vi "SV Aures Sharpness (Octave_2014) (1 Ch).vi"(0 "octave spectrum":T7={"nominal frequencies [Hz]"=[25.0, 31.5, 40.0, 50.0, 63.0, 80.0, 100.0, 125.0, 160.0, 200.0, 250.0, 315.0, 400.0, 500.0, 630.0, 800.0, 1000.0, 1250.0, 1600.0, 2000.0, 2500.0, 3150.0, 4000.0, 5000.0, 6300.0, 8000.0, 10000.0, 12500.0], "band power"=[-99.0, -99.0, -99.0, -99.0, -99.0, -99.0, -99.0, -99.0, -99.0, -99.0, -99.0, -99.0, -99.0, -99.0, 20.0, 40.0, 60.0, 40.0, 20.0, -99.0, -99.0, -99.0, -99.0, -99.0, -99.0, -99.0, -99.0, -99.0]} {"band power" format="%.2f"; "nominal frequencies [Hz]" format="%.2f"}, 1 "diffuse field":bool, 9 "octave info":T2={"standard"=enum."IEC 61260", "bandwidth"=enum."1/3 octave", "low band"=-16, "high band"=11, "weighting filter"=0, "dB reference"=2e-05, "dB On"=TRUE, "unit label"="Pa^2 rms|SV Units|dB ref 20u Pa", "channel name"="", "description"="", "engineering units"=2, "custom label"="", "spectrum type"=enum."power", "spectral density"=FALSE, "filters settled"=FALSE} {"engineering units" items=["custom..."=0, "V"=1, "A"=21, "C"=30, "pC"=31, "s"=32, "-"=29, "Pa"=2, "N"=20, "g"=3, "m/s^2"=4, "m/s"=5, "m"=6, "mm/s"=12, "mm"=13, "micron/s"=14, "micron"=15, "in/s^2"=7, "in/s"=8, "in"=9, "mil/s"=10, "mil"=11, "rad/s^2"=16, "rad/s"=17, "rad"=18, "deg/s^2"=26, "deg/s"=27, "deg"=28, "RPM"=22, "cycle/s^2"=23, "Hz"=24, "cycle"=25, "strain"=19]; "dB reference" format="%.2e"; "weighting filter" items=["Linear", "A-weighting", "B-weighting", "C-weighting", "ITU-R 468-4", "Dolby", "CCITT", "C-message", "Wb", "Wc", "Wd", "We", "Wf", "Wh", "Wj", "Wk", "Wm", "AES17 20 kHz lowpass", "AES17 40 kHz lowpass", "AES17 20 kHz highpass", "AES17 40 kHz highpass"]}, 11 "error in (no error)":errorcluster) -> (4 "specific sharpness":T6, 6 "sharpness [acum]":dbl format="%.2f", 10 "sharpness info":T1, 15 "error out":errorcluster)   [LabVIEW 2017, in "SoundVib_SoundQuality.lvlib"]
doc: "Computes sharpness from the sound pressure signal waveform, the 1/3-octave band spectrum calculated over the frequency range 25 Hz to 12.5 kHz, or the specific loudness that the SV Stationary Loudness VI returns. Wire data to the <B>sound pressure signal [Pa]</B> input to determine the polymorphic instance to use or manually select the instance."
uses:
  <vilib>/addons/Sound and Vibration/svt_Sound Quality/SoundVib_SoundQuality.lvlib
  <vilib>/addons/_NISVFA/_Shared subVIs/Controls/svc_Octave Info.ctl
  <vilib>/addons/_NISVFA/_Shared subVIs/Controls/svc_Octave Standard.ctl
  <vilib>/addons/_NISVFA/_Shared subVIs/Controls/svc_Weighting Filter Text Ring.ctl
  <vilib>/addons/_NISVFA/_Shared subVIs/Controls/svc_Engineering Units Text Ring.ctl
  <vilib>/addons/_NISVFA/_Shared subVIs/Controls/svc_SQ Info.ctl
  <vilib>/addons/Sound and Vibration/svt_Octave_2014 standard/SVT Octave Spectrum Conversion (1 Ch).vi
  <vilib>/addons/Sound and Vibration/svt_Octave/SoundVib_Octave_2014 standard.lvlib
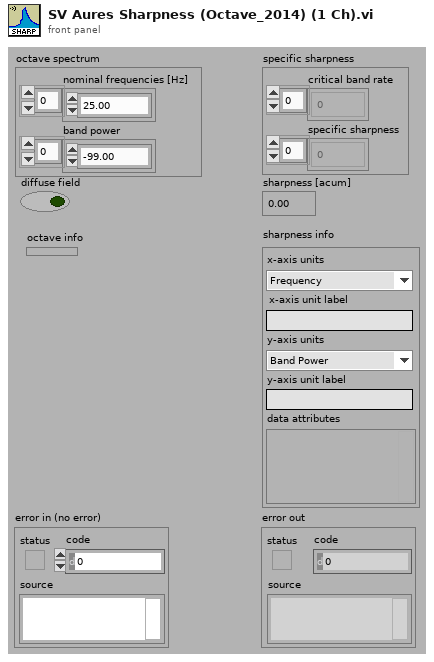
[diagram p1: front panel]
types:
  T1 = typedef "svc_SQ Info.ctl" = cluster{"x-axis units":enum16{"Frequency", "Critical Band", "Critical Band Rate"}, "x-axis unit label":string, "y-axis units":enum16{"Band Power", "Level", "Loudness", "Sharpness", "Roughness", "Fluctuation Strength", "Tonality"}, "y-axis unit label":string, "data attributes":variant}
  T2 = typedef "svc_Octave Info.ctl" = cluster{"standard":T3, "bandwidth":enum16{"1 octave", "1/3 octave", "1/6 octave", "1/12 octave", "1/24 octave"}, "low band":i32, "high band":i32, "weighting filter":T4, "dB reference":dbl, "dB On":bool, "unit label":string, "channel name":string, "description":string, "engineering units":T5, "custom label":string, "spectrum type":enum16{"power", "magnitude"}, "spectral density":bool, "filters settled":bool}
  T3 = typedef "svc_Octave Standard.ctl" = enum16{"ANSI S1.11", "IEC 61260"}
  T4 = typedef "svc_Weighting Filter Text Ring.ctl" = u16
  T5 = typedef "svc_Engineering Units Text Ring.ctl" = u16
  T6 = cluster{"critical band rate":dbl[], "specific sharpness":dbl[]}
  T7 = cluster{"nominal frequencies [Hz]":dbl[], "band power":dbl[]}
  T8 = cluster{"linear/dB":enum16{"no change", "linear", "dB"}, "dB reference (0: no change)":dbl, "power/magnitude":enum16{"no change", "power", "magnitude"}, "spectral density":enum16{"no change", "spectrum", "spectral density"}}
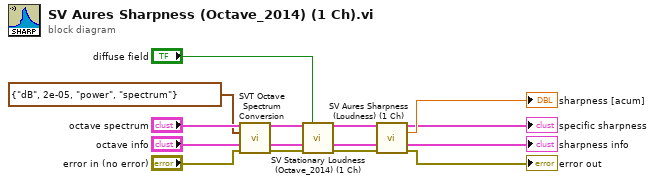
[diagram p0: block diagram]
diagram:
  n1 = call-poly <vilib>:"SVT Octave Spectrum Conversion.vi"("octave spectrum"="octave spectrum", "desired scaling"=T8 {"linear/dB"=enum."dB", "dB reference (0: no change)"=2e-05, "power/magnitude"=enum."power", "spectral density"=enum."spectrum"}, "octave info in"="octave info", "error in (no error)"="error in (no error)") -> ("converted octave spectrum"=w6:T7, "octave info out"=w2:T2, "error out"=w3:errorcluster)  [unwired: 8 in, 1 out]
  n2 = call <vilib>:"SV Stationary Loudness (Octave_2014) (1 Ch).vi"("octave spectrum"=w6, "diffuse field"="diffuse field", "octave info"=w2, "error in (no error)"=w3) -> ("specific loudness"=w12:cluster{dbl[], "Nm":dbl[]}, "loudness info"=w13:T1, "error out"=w14:errorcluster)  [unwired: 7 in, 2 out]
  n3 = call <vilib>:"SV Aures Sharpness (Loudness) (1 Ch).vi"("specific loudness"=w12, "loudness info"=w13, "error in (no error)"=w14) -> ("specific sharpness"=→"specific sharpness":T6, "sharpness [acum]"=→"sharpness [acum]":dbl, "sharpness info"=→"sharpness info":T1, "error out"=→"error out":errorcluster)  [unwired: 9 in]
